vi "Lockin.DAQ.Create.AO Task.vi"(8 "error in (no error)":errorcluster, 11 "Lockin.DAQ":refnum<class "Lockin.DAQ.lvclass">) -> (0 "error out":errorcluster, 3 "Lockin.DAQ":refnum<class "Lockin.DAQ.lvclass">)   [LabVIEW 2016, in "Lockin.DAQ.lvclass"]
uses:
  Lockin.DAQ.lvclass
  Lockin.DAQ.lvclass/Lockin.DAQ.ctl
  <vilib>/DAQmx/create/channels.llb/DAQmx Create Channel (AO-Voltage-Basic).vi
  <resource>/objmgr/daqmx.rc
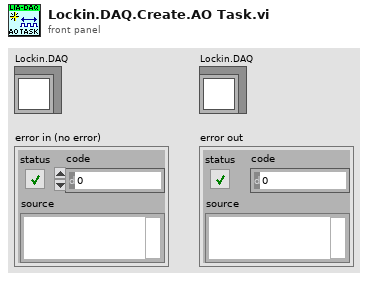
[diagram p1: front panel]
types:
  T1 = typedef "Lockin.DAQ.lvclass/AO.config-array.ctl" = T2[]
  T2 = typedef "Lockin.DAQ.lvclass/AO.config-cluster.ctl" = cluster{"AO.channels":tag, "AO.Range":T3, "output terminal configuration":i32, "DAQ Type":T4}
  T3 = typedef "Lockin.DAQ.lvclass/446xAO-enum.ctl" = enum16{"±0.1 V", "±1.0 V", "±10.0 V"}
  T4 = typedef "Lockin.DAQ.lvclass/DAQType-enum.ctl" = enum16{"None", "USB 4431", "PXI 446x"}
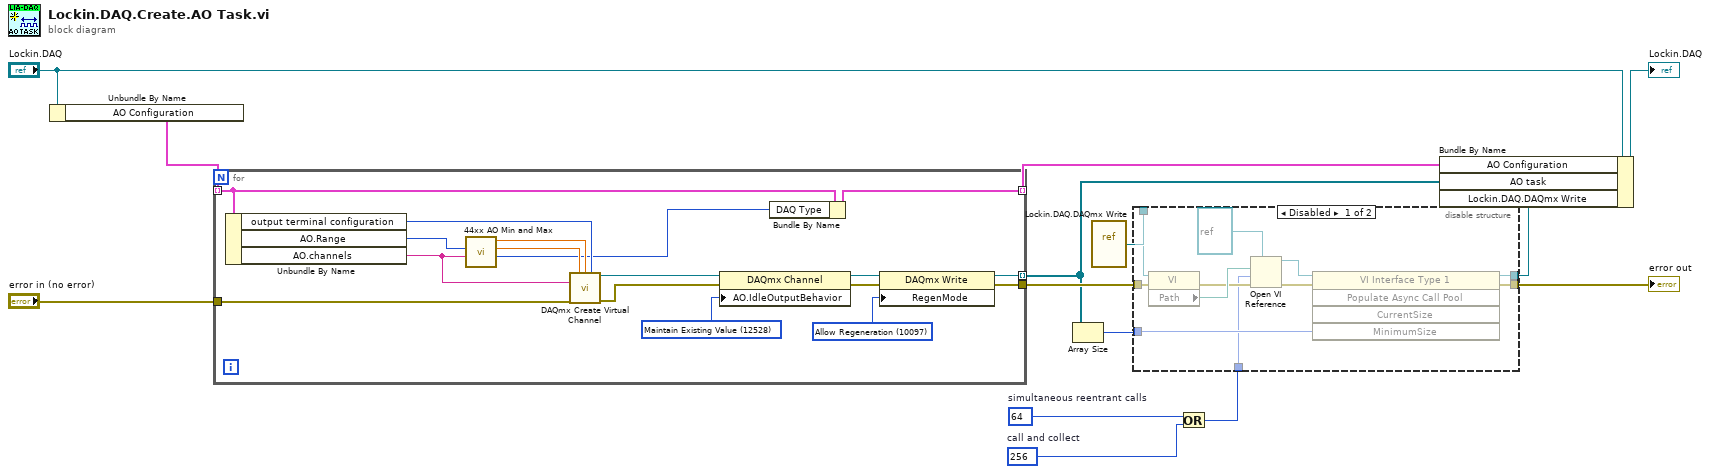
[diagram p0: block diagram]
diagram:
  w2 = 64  # simultaneous reentrant calls
  w3 = 256  # call and collect
  n1 = Unbundle By Name("Lockin.DAQ") -> ("AO Configuration"=w13:T1)
  n2 = for {
    tunnel: "error in (no error)" -> [w28]
    tunnel: [w16] -> w7
    tunnel: w13 -> [w15] mode=indexing
    tunnel: [w20] -> w11 mode=indexing
    tunnel: [w22] -> w5 mode=indexing
    w17 = 10097 items=["Allow Regeneration"=10097, "Do Not Allow Regeneration"=10158] ("RegenMode")
    w18 = 12528 items=["Zero Volts"=12526, "High-Impedance"=12527, "Maintain Existing Value"=12528] ("AO.IdleOutputBehavior")
    n3 = Unbundle By Name(w15) -> ("output terminal configuration"=w24:i32, "AO.Range"=w23:T3, "AO.channels"=w25:tag)
    n4 = call "44xx AO Min and Max.vi"("AO.channels"=w25, "AO.Range"=w23) -> ("DAQ Type"=w21:T4, "AO.max"=w27:dbl, "AO.min"=w26:dbl)  [unwired: 7 in]
    n5 = call-poly <vilib>:"DAQmx Create Virtual Channel.vi"("maximum value"=w27, "minimum value"=w26, "output terminal configuration"=w24, "physical channels"=w25, "error in"=w28) -> ("task out"=w31:refnum<k21>, "error out"=w19:errorcluster)  [unwired: 9 in]
    n6 = property class="DAQmx Channel"(reference=w31, error in=w19, "AO.IdleOutputBehavior"=w18) -> (reference out=w30:refnum<k21>, error out=w29:errorcluster)
    n7 = Bundle By Name(cluster=w15, "DAQ Type"=w21) -> (w20:T2)
    n8 = property class="DAQmx Write"(reference=w30, error in=w29, "RegenMode"=w17) -> (reference out=w22:refnum<k21>, error out=w16:errorcluster)
  }
  n9 = Array Size(array=w5) -> (size(s)=w8:i32)
  n10 = vi-ref "Lockin.DAQ.DAQmx Write.vi"() -> (w9:refnum<vi>)
  n11 = Or(x=w2, y=w3) -> (x .or. y?=w1:i32)
  n12 = disable-structure shown="Disabled" {
    disable-tunnel: w9 -> [w42 _]
    disable-tunnel: w8 -> [w36 _]
    disable-tunnel: w7 -> [w35 w43]
    disable-tunnel: [w34 w43] -> w6
    disable-tunnel: [w33 _] -> w4
    disable-tunnel: w1 -> [w32 _]
    frame Disabled {
      n13 = property class="VI"(reference=w42, error in=w35) -> (error out=w40:errorcluster, "Path"=w41:path)  [unwired: 1 out]
      n14 = Open VI Reference(type specifier VI Refnum (for type only)=refnum<vi> refnum, vi path=w41, options=w32, error in (no error)=w40) -> (vi reference=w38:refnum<vi>, error out=w37:errorcluster)  [unwired: 2 in]
      n15 = invoke class="VI Interface Type 1" method="Populate Async Call Pool"(reference=w38, error in=w37, "MinimumSize"=w36) -> (reference out=w33:refnum<vi>, error out=w34:errorcluster)  [unwired: 2 in, 3 out]
    }
    frame Enabled {
    }
  }
  "error out" <- w6
  n16 = Bundle By Name(cluster="Lockin.DAQ", "AO Configuration"=w11, "AO task"=w5, "Lockin.DAQ.DAQmx Write"=w4) -> (→"Lockin.DAQ":refnum<class "Lockin.DAQ.lvclass">)
